vi "data log_append.vi"(9 "data":dbl[](array[numeric]) format="%0.2f", 10 "current time":timestamp, 11 "Data Log In":T1) -> (3 "Data Log Out":T1)   [LabVIEW 2025]
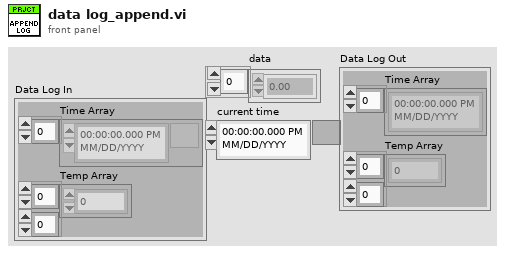
[diagram p1: front panel]
types:
  T1 = cluster{"Time Array":timestamp[], "Temp Array":dbl[][]}
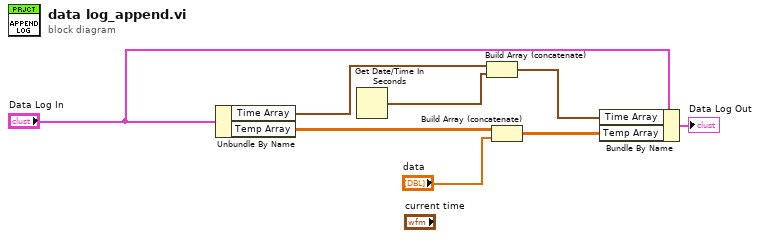
[diagram p0: block diagram]
diagram:
  n1 = Unbundle By Name("Data Log In") -> ("Time Array"=w4:timestamp[], "Temp Array"=w8:dbl[][])
  n2 = Get Date/Time In Seconds() -> (seconds since 1Jan1904=w3:timestamp)
  n3 = Build Array (concatenate)(w4, w3) -> (w2:timestamp[])
  n4 = Build Array (concatenate)(w8, "data") -> (w5:dbl[][])
  n5 = Bundle By Name(cluster="Data Log In", "Time Array"=w2, "Temp Array"=w5) -> (→"Data Log Out":T1)
